vi "Test SFOAE Stimuli.vi"() -> ()   [LabVIEW 2015]
uses:
  Typedefs/SFOAE-Stimulus Parameters.ctl
  Typedefs/SFOAE-Sweep Params.ctl
  Utility VIs/Math VIs/FFT x(t) to dB,Degrees (1D).vi
panel:
  out "Magnitude":cluster{"Array":dbl[], "Array":dbl[]}[](graph)
  in  "Cal File":path=path "C:/Experiment VIs/Cochlear Function Test Suite/LV Source/SFOAE VIs/Test VIs/dummy.calib"
  out "XY Graph":cluster{"Array":dbl[], "Array":dbl[]}[](graph)
  in  "Fs (Hz)":dbl=100000.0
  in  "SFOAE Stim":T1={"Ear"=enum."Right", "Sweep"={"Type"=enum."Linear", "Fmin (kHz)"=4.0, "Fmax (kHz)"=44.0, "Rate"=5.0, "Ramp (ms)"=5.0, "Drain (ms)"=20.0}, "Suppressor"={"Delta"=50.0, "Ratio"=0.0, "Use ratio"=FALSE}, "Concurrent"={"Nsweeps"=4, "Overlap"=0.0}, "Ls (dB SPL)"=-23.0, "Lp (dB SPL)"={"Min"=-20.0, "Max"=-20.0, "Step"=5.0}}
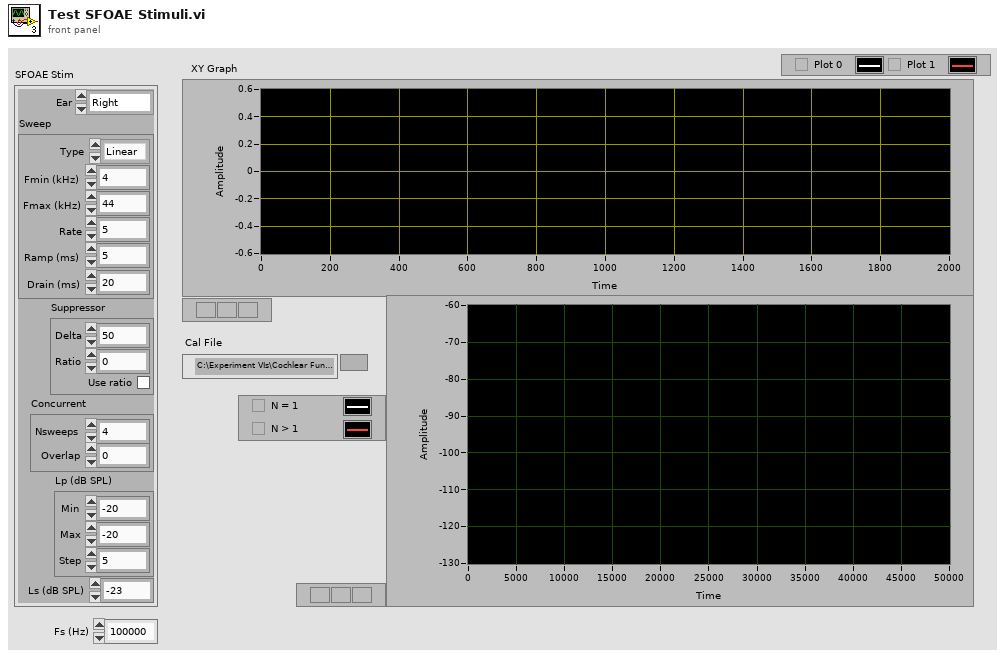
[diagram p1: front panel]
types:
  T1 = typedef "SFOAE-Stimulus Parameters.ctl" = cluster{"Ear":enum16{"Right", "Left"}, "Sweep":T2, "Suppressor":cluster{"Delta":dbl, "Ratio":dbl, "Use ratio":bool}, "Concurrent":cluster{"Nsweeps":i32, "Overlap":dbl}, "Ls (dB SPL)":dbl, "Lp (dB SPL)":cluster{"Min":dbl, "Max":dbl, "Step":dbl}}
  T2 = typedef "SFOAE-Sweep Params.ctl" = cluster{"Type":enum16{"Linear", "Log"}, "Fmin (kHz)":dbl, "Fmax (kHz)":dbl, "Rate":dbl, "Ramp (ms)":dbl, "Drain (ms)":dbl}
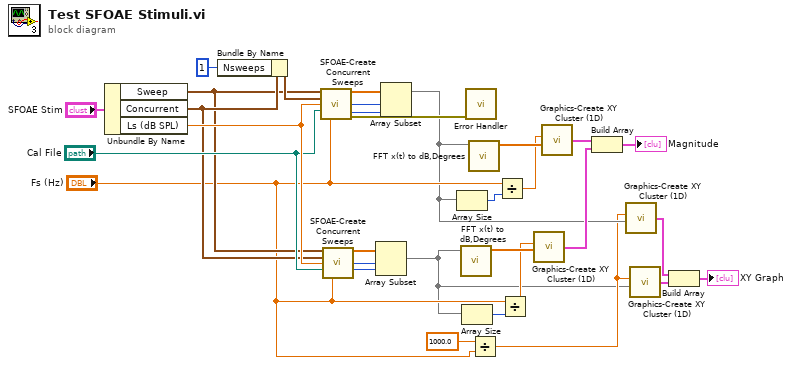
[diagram p0: block diagram]
diagram:
  n1 = Unbundle By Name("SFOAE Stim") -> ("Sweep"=w8:T2, "Concurrent"=w9:cluster{"Nsweeps":i32, "Overlap":dbl}, "Ls (dB SPL)"=w11:dbl)
  n2 = Bundle By Name(cluster=w9, "Nsweeps"=1) -> (w18:cluster{"Nsweeps":i32, "Overlap":dbl})
  n3 = call "SFOAE-Create Concurrent Sweeps.vi"("Sweep"=w8, "Concurrent"=w18, "Level (dB SPL)"=w11, "Cal File"="Cal File", "Fs (Hz)"="Fs (Hz)") -> ("sweep"=w15:dbl[], "offset"=w13:i32, "nfft"=w12:i32, "error out"=w31:errorcluster)  [unwired: 7 in]
  n4 = call "SFOAE-Create Concurrent Sweeps.vi"("Sweep"=w8, "Concurrent"=w9, "Level (dB SPL)"=w11, "Cal File"="Cal File", "Fs (Hz)"="Fs (Hz)") -> ("sweep"=w2:dbl[], "offset"=w24:i32, "nfft"=w23:i32)  [unwired: 7 in, 1 out]
  n5 = Array Subset(array=w2, index=w24, length=w23) -> (w1:dbl[])
  n6 = Array Subset(array=w15, index=w13, length=w12) -> (w6:dbl[])
  n7 = Array Size(array=w6) -> (size(s)=w16:i32)
  n8 = call-poly "FFT x(t) to dB,Degrees.vi"("X"=w1) -> ("+Freq. Mag of FFT (dB rms)"=w28:dbl[])  [unwired: 8 in, 2 out]
  n9 = Array Size(array=w1) -> (size(s)=w3:i32)
  n10 = call "Error Handler.vi"("error in (no error)"=w31) -> ()  [unwired: 13 in, 2 out]
  n11 = call-poly "FFT x(t) to dB,Degrees.vi"("X"=w6) -> ("+Freq. Mag of FFT (dB rms)"=w27:dbl[])  [unwired: 8 in, 2 out]
  n12 = Divide(x=1000.0, y="Fs (Hz)") -> (x/y=w5:dbl)
  n13 = Divide(x="Fs (Hz)", y=w16) -> (x/y=w26:dbl)
  n14 = Divide(x="Fs (Hz)", y=w3) -> (x/y=w25:dbl)
  n15 = call "Graphics-Create XY Cluster (1D).vi"("Array"=w28, "dx"=w25) -> ("XY cluster"=w14:cluster{"Array":dbl[], "Array":dbl[]})  [unwired: 2 in]
  n16 = call "Graphics-Create XY Cluster (1D).vi"("Array"=w27, "dx"=w26) -> ("XY cluster"=w30:cluster{"Array":dbl[], "Array":dbl[]})  [unwired: 2 in]
  n17 = Build Array(w30, w14) -> (→"Magnitude":cluster{"Array":dbl[], "Array":dbl[]}[])
  n18 = call "Graphics-Create XY Cluster (1D).vi"("Array"=w6, "dx"=w5) -> ("XY cluster"=w4:cluster{"Array":dbl[], "Array":dbl[]})  [unwired: 2 in]
  n19 = call "Graphics-Create XY Cluster (1D).vi"("Array"=w1, "dx"=w5) -> ("XY cluster"=w22:cluster{"Array":dbl[], "Array":dbl[]})  [unwired: 2 in]
  n20 = Build Array(w4, w22) -> (→"XY Graph":cluster{"Array":dbl[], "Array":dbl[]}[])
